vi "Is DVR Valid.vi"(8 "dvr error in":errorcluster, 11 "dvr valid in":bool) -> (3 "dvr valid out":bool)   [LabVIEW 2020, in "Measurement Plugin Session Management V1.lvlib" / "Session Reservation.lvclass"]
uses:
  Session Reservation.lvclass
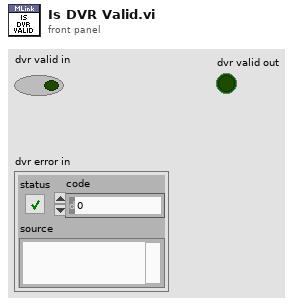
[diagram p1: front panel]
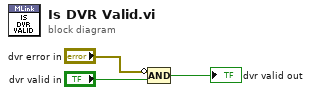
[diagram p0: block diagram]
diagram:
  n1 = Compound Arithmetic op=AND(invert "dvr error in", "dvr valid in") -> (→"dvr valid out":bool)
